vi "RIMAS Detector FITS hdr update field poly.vi"   [LabVIEW 2020]
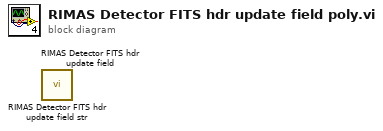
[diagram p0: block diagram]
diagram:
  n1 = call "RIMAS Detector FITS hdr update field str.vi"() -> ()  [unwired: 10 in, 2 out]
  n2 = call "RIMAS Detector FITS hdr update field.vi"() -> ()  [unwired: 10 in, 2 out]
